vi "Form Line.vi"(2 "State":string, 3 "Element":string) -> (0 "New State":string)   [LabVIEW 2020, in "Examples.lvlib"]
uses:
  Examples.lvlib
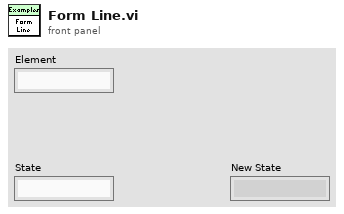
[diagram p1: front panel]
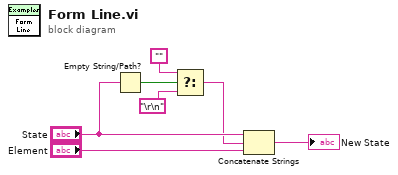
[diagram p0: block diagram]
diagram:
  n1 = Empty String/Path?(string/path="State") -> (empty?=w4:bool)
  n2 = Select(t="", s=w4, f="\r\n") -> (s? t:f=w1:string)
  n3 = Concatenate Strings("State", w1, "Element") -> (→"New State":string)
